vi "Waveform Output.vi"(8 "error in (no error)":errorcluster, 11 "Node Ptr":T1 format="%.0x") -> (0 "error out":errorcluster)   [LabVIEW 2026, in "FPGA Addon System Explorer.lvlib"]
uses:
  FPGA Addon System Explorer.lvlib
  <vilib>/NI VeriStand/Custom Device API/Custom Device Item Ref.ctl
  NationalInstruments.VeriStand.SystemStorageUI
  Addon Shared/SubVIs/Constants.vi
  <vilib>/NI VeriStand/Custom Device API/Get Item Property (Dependent Node Pointer).vi
  <vilib>/NI VeriStand/Custom Device API/Set Item Property (Dependent Node Pointer).vi
  C:/Users/Administrator/Desktop/Jatin/All DNC DLLs/NationalInstruments.VeriStand.SystemStorage.dll
  Jatin/All DNC DLLs/NationalInstruments.VeriStand.SystemStorage.dll
  C:/Users/Administrator/Desktop/Jatin/All DNC DLLs/NationalInstruments.VeriStand.SystemStorageUI.dll
  Jatin/All DNC DLLs/NationalInstruments.VeriStand.SystemStorageUI.dll
  <vilib>/NI VeriStand/Custom Device API/Custom Device API.lvlib
  <vilib>/NI VeriStand/UI Controls/Single Node Browser/NI_VS UI Single Node Browser.lvlib
  Addon Shared/FPGA Addon Shared.lvlib
panel:
  out "Original Name":string
  in  "Source Waveform":refnum<k24>(container)
  in  "Header":cluster{"Section Name":string}={"Section Name"="Wavefrom Output Settings"}
  in  "Description":string
  in  "Name":string
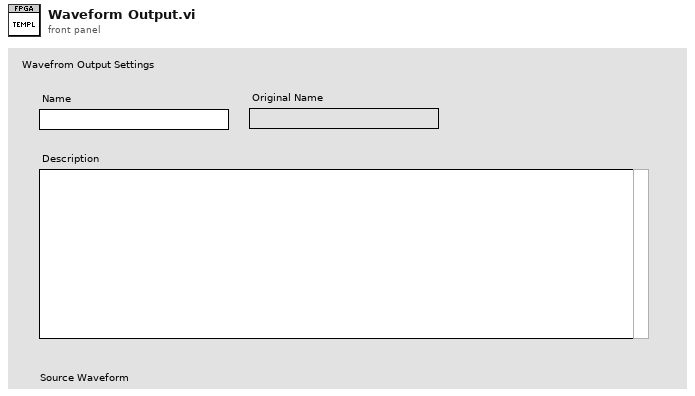
[diagram p1: front panel]
types:
  T1 = typedef "Custom Device API.lvlib/Custom Device Item Ref.ctl" = u64
  T2 = typedef "Custom Device API.lvlib/Custom Device Pointer.ctl" = refnum<k39>
  T3 = typedef "Custom Device API.lvlib/Custom Device Item Info.ctl" = cluster{"Name":string, "Is Channel":bool, "GUID":string, "Is Waveform":bool}
  T4 = typedef "NI_VS UI Single Node Browser.lvlib/Callback Type.ctl" = cluster{"Net Callbacks":refnum<k27>[], "Event":refnum<user-event>}
  T5 = typedef "Custom Device API.lvlib/Custom Device Commands.ctl" = enum16{"Default", "Item renamed", "Shutdown", "Dynamic button pressed"}
  T6 = typedef "NI_VS UI Single Node Browser.lvlib/Node Ref.ctl" = refnum<k39>
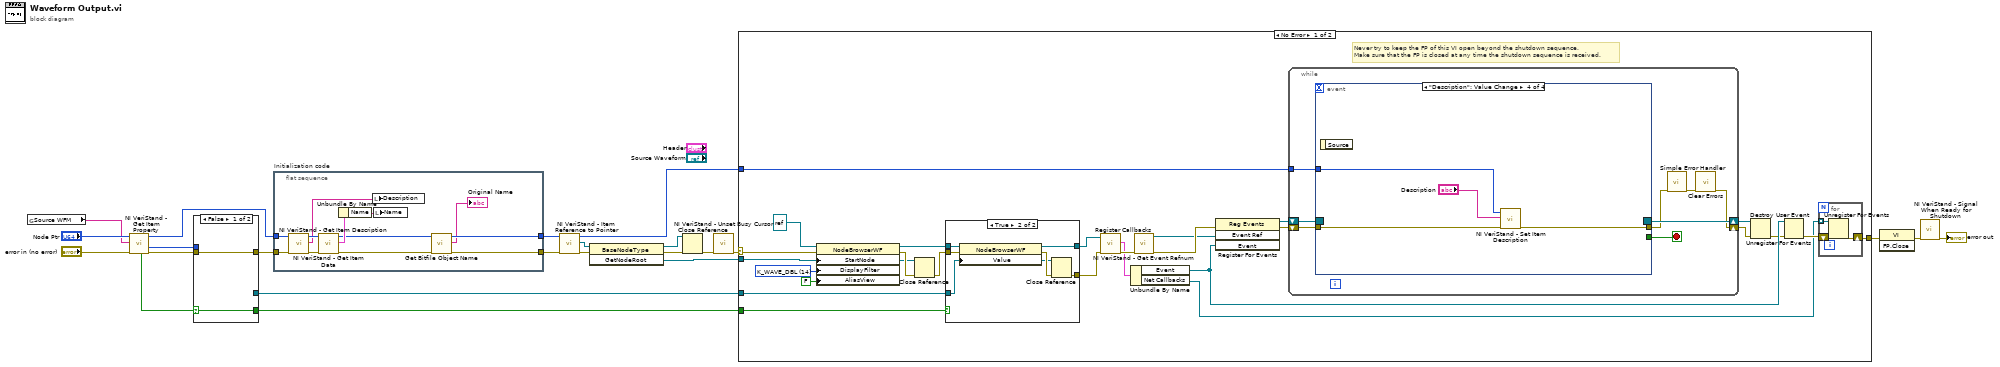
[diagram p0: block diagram]
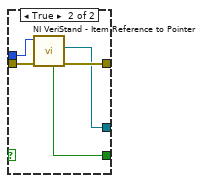
[diagram p2: hidden frame]
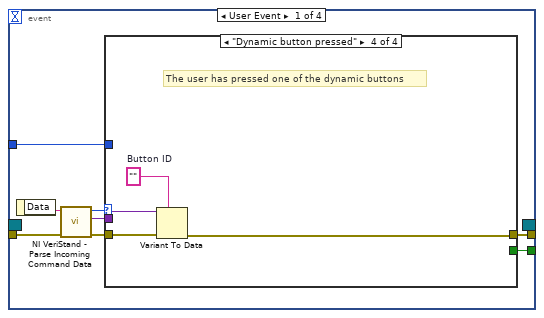
[diagram p4: hidden frame]
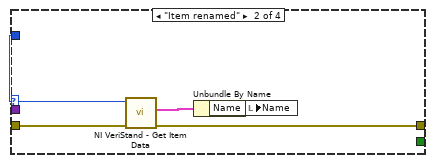
[diagram p6: hidden frame]
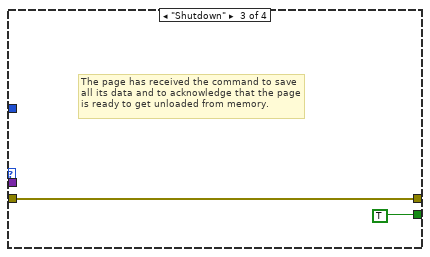
[diagram p7: hidden frame]
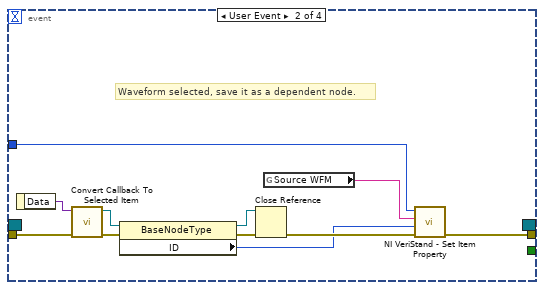
[diagram p8: hidden frame]
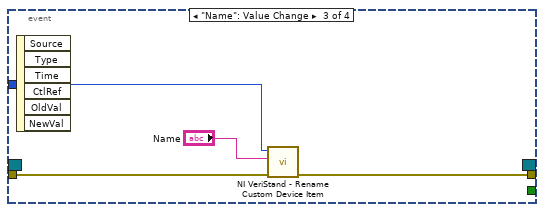
[diagram p9: hidden frame]
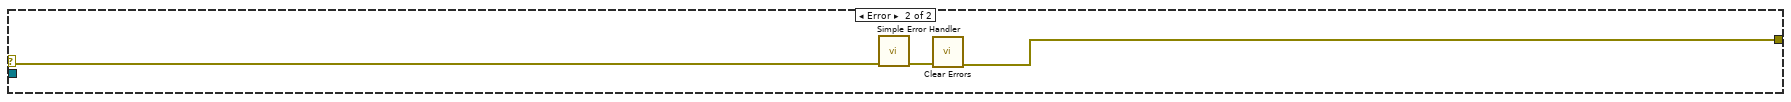
[diagram p10: hidden frame]
diagram:
  n1 = global read "Constants.vi" "Source WFM"() -> (w1:string)
  n2 = call-poly <vilib>:"NI VeriStand - Get Item Property.vi"("error in (no error)"="error in (no error)", "Property Name"=w1, "Item Ref in"="Node Ptr") -> ("error out"=w12:errorcluster, "Dependent Node Ref"=w11:T1, "Item Ref out"=w5:T1, "Found"=w10:bool)  [unwired: 5 in]
  n3 = case shown="False" w10 {
    selector: w10 -> [w24 _]
    tunnel: [w25 w30] -> w6
    tunnel: [_ w29] -> w13
    tunnel: w12 -> [w25 w28]
    tunnel: w11 -> [_ w27]
    tunnel: [w24 w26] -> w9
    frame False {
    }
    frame True {
      n4 = call <vilib>:"NI VeriStand - Item Reference to Pointer.vi"("error in (no error)"=w28, "Item Ref in"=w27) -> ("error out"=w30:errorcluster, "Node Pointer"=w29:T2, "Found"=w26:bool)  [unwired: 6 in, 1 out]
    }
  }
  n5 = flat-sequence "Initialization code" {
    tunnel: w6 -> [w41]
    tunnel: w5 -> [w40]
    tunnel: [w34] -> w4
    tunnel: [w32] -> w3
    frame #0 {
      n6 = call <vilib>:"NI VeriStand - Get Item Description.vi"("error in (no error)"=w41, "Item Ref in"=w40) -> ("error out"=w38:errorcluster, "Description"=w39:string, "Item Ref out"=w42:T1)  [unwired: 7 out]
      n7 = call <vilib>:"NI VeriStand - Get Item Data.vi"("error in (no error)"=w38, "Item Ref in"=w42) -> ("error out"=w35:errorcluster, "Item Info"=w37:T3, "Item Ref out"=w33:T1)  [unwired: 7 out]
      n8 = Unbundle By Name(w37) -> ("Name"=w36:string)
      n9 = local write "Description"(w39) -> ()
      n10 = local write "Name"(w36) -> ()
      n11 = call "Get Bitfile Object Name.vi"("error in (no error)"=w35, "Item Ref in"=w33) -> ("error out"=w34:errorcluster, "Value"=→"Original Name":string, "Item Ref out"=w32:T1)  [unwired: 7 in]
    }
  }
  n12 = call <vilib>:"NI VeriStand - Item Reference to Pointer.vi"("error in (no error)"=w4, "Item Ref in"=w3) -> ("error out"=w18:errorcluster, "Node Pointer"=w19:T2, "Item Ref out"=w20:T1)  [unwired: 6 in, 1 out]
  n13 = invoke class="BaseNodeType" method="GetNodeRoot"(reference=w19, error in=w18) -> (reference out=w14:T2, error out=w15:errorcluster, "GetNodeRoot"=w17:refnum<k39>)  [unwired: 1 in]
  n14 = Close Reference(reference=w14, error in (no error)=w15) -> (error out=w16:errorcluster)
  n15 = call <vilib>:"NI VeriStand - Unset Busy Cursor.vi"("error in (no error)"=w16) -> ("error out"=w21:errorcluster)  [unwired: 10 out]
  n16 = case shown="No Error" w21 {
    selector: w21 -> [w57 w129]
    tunnel: [w51 w127] -> w23
    tunnel: w20 -> [w62 _]
    tunnel: w17 -> [w55 _]
    tunnel: w13 -> [w45 _]
    tunnel: w9 -> [w44 _]
    frame No Error {
      w59 = u8 14 items=["K_CHAN_R", "K_CHAN_W", "K_CHAN_RW", "K_CHAN_VOLT", "K_CHAN_FAULT", "K_ALL", "K_CUSTOM", "K_CHAN_R_VIS", "K_CHAN_W_VIS", "K_CHAN_RW_VIS", "K_CHAN_VOLT_VIS", "K_CHAN_FAULT_VIS", "K_WAVE", "K_WAVE_VIS", "K_WAVE_DBL", "K_WAVE_CDB", "K_WAVE_DBL_VIS", "K_WAVE_CDB_VIS"] ("DisplayFilter")
      # "Never try to keep the FP of this VI open beyond the shutdown sequence.\nMake sure that the FP is closed at any time the shutdown sequence is received."
      n17 = property class="NodeBrowserWF"(reference=refnum<k39> refnum, error in=w57, "StartNode"=w55, "DisplayFilter"=w59, "AliasView"=FALSE) -> (reference out=w47:refnum<k39>, error out=w56:errorcluster)
      n18 = Close Reference(reference=w55, error in (no error)=w56) -> (error out=w48:errorcluster)
      n19 = case shown="True" w44 {
        tunnel: [w69 w76] -> w49
        tunnel: w48 -> [w69 w75]
        tunnel: w47 -> [w70 w74]
        tunnel: [w70 w72] -> w46
        tunnel: w45 -> [_ w71]
        frame False {
        }
        frame True {
          n20 = property class="NodeBrowserWF"(reference=w74, error in=w75, "Value"=w71) -> (reference out=w72:refnum<k39>, error out=w73:errorcluster)
          n21 = Close Reference(reference=w71, error in (no error)=w73) -> (error out=w76:errorcluster)
        }
      }
      n22 = call <vilib>:"Register Callbacks.vi"("error in (no error)"=w49, "Single Node Browser"=w46) -> ("error out"=w61:errorcluster, "Callbacks"=w60:T4)  [unwired: 7 in, 1 out]
      n23 = Unbundle By Name(w60) -> ("Event"=w54:refnum<user-event>, "Net Callbacks"=w50:refnum<k27>[])
      n24 = call <vilib>:"NI VeriStand - Get Event Refnum.vi"("error in (no error)"=w61) -> ("error out"=w68:errorcluster, "Event Ref"=w65:refnum<user-event>)  [unwired: 9 out]
      n25 = register-events(error in=w68, w65, w54) -> (reference out=w63:refnum<event-registration>, error out=w64:errorcluster)  [unwired: 1 in]
      n26 = while {
        tunnel: w62 -> [w83]
        shift-right: [w80] -> w66
        shift-left: w64 -> [w86]
        shift-right: [w87] -> w67
        shift-left: w63 -> [w85]
        stop <- w84 stop-if-true
        n27 = event shown="[3] \"Description\": Value Change" {
          selector: w85 -> [_ _ _ _]
          dyn-events: [_ _ _ _] -> w87
          timeout: _ -> [_ _ _ _]
          tunnel: w86 -> [w95 w118 w122 w125]
          tunnel: [w91 _ _ _] -> w84
          tunnel: [w90 w111 w121 w124] -> w82
          tunnel: w83 -> [w89 w112 w120 w126]
          event User Event {
            n28 = event-data() -> ("Data"=w94:string)  [unwired: 1 out]
            n29 = call <vilib>:"NI VeriStand - Parse Incoming Command Data.vi"("error in (no error)"=w95, "Incoming data"=w94) -> ("error out"=w93:errorcluster, "Outgoing data"=w88:variant, "Action"=w92:T5)  [unwired: 7 out]
            n30 = case shown="\"Dynamic button pressed\"" w92 {
              tunnel: w93 -> [w96 w101 w102 w107]
              tunnel: [_ _ TRUE _] -> w91
              tunnel: [w96 w98 w102 w104] -> w90
              tunnel: w89 -> [_ w100 _ _]
              tunnel: w88 -> [_ _ _ w106]
              frame "Default", Default {
              }
              frame "Item renamed" {
                n31 = call <vilib>:"NI VeriStand - Get Item Data.vi"("error in (no error)"=w101, "Item Ref in"=w100) -> ("error out"=w98:errorcluster, "Item Info"=w99:T3)  [unwired: 8 out]
                n32 = Unbundle By Name(w99) -> ("Name"=w97:string)
                n33 = local write "Name"(w97) -> ()
              }
              frame "Shutdown" {
                # "The page has received the command to save all its data and to acknowledge that the page is ready to get unloaded from memory."
              }
              frame "Dynamic button pressed" {
                w105 = ""  # Button ID
                # "The user has pressed one of the dynamic buttons"
                n34 = Variant To Data(error in=w107, type=w105, Variant=w106) -> (error out=w104:errorcluster)  [unwired: 1 out]
              }
            }
          }
          event User Event {
            # "Waveform selected, save it as a dependent node."
            n35 = event-data() -> ("Data"=w117:variant)  [unwired: 1 out]
            n36 = call <vilib>:"Convert Callback To Selected Item.vi"("error in"=w118, "Data"=w117) -> ("error out"=w116:errorcluster, "Selected Item"=w115:T6)  [unwired: 8 in]
            n37 = property class="BaseNodeType"(reference=w115, error in=w116) -> (reference out=w113:T6, error out=w114:errorcluster, "ID"=w109:u64)
            n38 = Close Reference(reference=w113, error in (no error)=w114) -> (error out=w110:errorcluster)
            n39 = global read "Constants.vi" "Source WFM"() -> (w108:string)
            n40 = call-poly <vilib>:"NI VeriStand - Set Item Property.vi"("error in (no error)"=w110, "Dependent Node Ref"=w109, "Property Name"=w108, "Item Ref in"=w112) -> ("error out"=w111:errorcluster)  [unwired: 5 in, 2 out]
          }
          event "Name": Value Change {
            n41 = event-data() -> ()  [unwired: 7 out]
            n42 = call <vilib>:"NI VeriStand - Rename Custom Device Item.vi"("error in (no error)"=w122, "New Name"="Name", "Item Ref in"=w120) -> ("error out"=w121:errorcluster)  [unwired: 1 in, 7 out]
          }
          event "Description": Value Change {
            n43 = event-data() -> ()  [unwired: 2 out]
            n44 = call <vilib>:"NI VeriStand - Set Item Description.vi"("error in (no error)"=w125, "Description"="Description", "Item Ref in"=w126) -> ("error out"=w124:errorcluster)  [unwired: 8 out]
          }
        }
        n45 = call <vilib>:"Simple Error Handler.vi"("error in (no error)"=w82) -> ("error out"=w81:errorcluster)  [unwired: 1 in, 7 out]
        n46 = call <vilib>:"Clear Errors.vi"("error in (no error)"=w81) -> ("error out"=w80:errorcluster)  [unwired: 1 in, 5 out]
      }
      n47 = Unregister For Events(event registration refnum=w67, error in=w66) -> (error out=w53:errorcluster)
      n48 = Destroy User Event(user event=w54, error in=w53) -> (error out=w52:errorcluster)
      n49 = for {
        tunnel: w50 -> [w77] mode=indexing
        shift-right: [w78] -> w51
        shift-left: w52 -> [w79]
        n50 = Unregister For Events(event registration refnum=w77, error in=w79) -> (error out=w78:errorcluster)
      }
    }
    frame Error {
      n51 = call <vilib>:"Simple Error Handler.vi"("error in (no error)"=w129) -> ("error out"=w128:errorcluster)  [unwired: 1 in, 7 out]
      n52 = call <vilib>:"Clear Errors.vi"("error in (no error)"=w128) -> ("error out"=w127:errorcluster)  [unwired: 1 in, 5 out]
    }
  }
  n53 = invoke class="VI" method="FP.Close"(error in=w23) -> (error out=w22:errorcluster)  [unwired: 2 in, 2 out]
  n54 = call <vilib>:"NI VeriStand - Signal When Ready for Shutdown.vi"("error in (no error)"=w22) -> ("error out"=→"error out":errorcluster)  [unwired: 10 out]
